vi "user initialization.vi"(8 "error in":errorcluster, 10 "configuration in":refnum<class "control module configuration.lvclass">, 11 "fixed channel runtime in":refnum<class "AppStateMachine runtime.lvclass">) -> (0 "error out":errorcluster, 3 "fixed channel runtime out":refnum<class "AppStateMachine runtime.lvclass">)   [LabVIEW 2017, in "AppStateMachine runtime.lvclass"]
uses:
  AppStateMachine runtime.lvclass
  <vilib>/NI/DCAF/Tag Editor Core/control module/configuration/control module configuration.lvclass
  <vilib>/NI/DCAF/addons/InstructionFrameworkSupport/FPGA_FGV_action.ctl
  <vilib>/userdefined/High Color/nirio_resource_hc.ctl
  StateId.ctl
  State.ctl
  LED_Color.ctl
  AppStateMachine runtime.lvclass/AppStateMachine runtime.ctl
  <vilib>/NI/DCAF/Tag Editor Core/control module/runtime/control module runtime.lvclass
  <vilib>/NI/NI JSONRPC Server Framework/Classes/Server/JSONRPC Server.lvclass
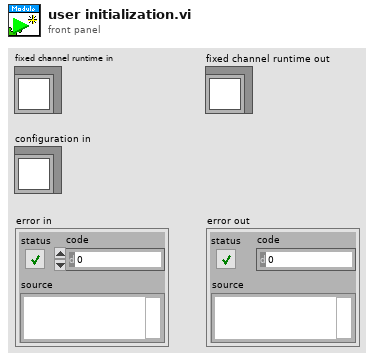
[diagram p1: front panel]
types:
  T1 = typedef "AppStateMachine runtime.lvclass/State.ctl" = cluster{"StateId":T2, "LED_Enable":bool, "LED_BlinksPerCycle":i32, "LED_Color":T3}
  T2 = typedef "AppStateMachine runtime.lvclass/StateId.ctl" = enum16{"Initialize", "Idle", "SafeState", "UnrecoverableSafeState"}
  T3 = typedef "AppStateMachine runtime.lvclass/LED_Color.ctl" = enum16{"Green", "Yellow"}
  T4 = typedef "nirio_resource_hc.ctl" = tag
  T5 = typedef "FPGA_FGV_action.ctl" = enum16{"get FPGA", "set FPGA", "Close"}
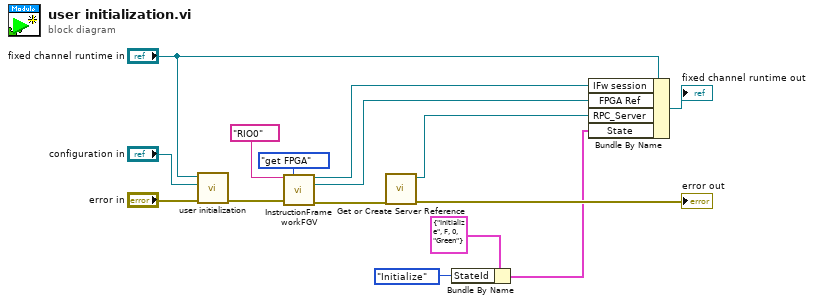
[diagram p0: block diagram]
diagram:
  n1 = call-parent "user initialization.vi"("error in"="error in", "configuration in"="configuration in", "fixed channel runtime in"="fixed channel runtime in") -> ("error out"=w13:errorcluster)  [unwired: 7 in, 1 out]
  n2 = call <vilib>:"InstructionFrameworkFGV.vi"("RIO resource"=T4 "RIO0", "Action"=FPGA_FGV_action."get FPGA", "error in"=w13) -> ("session out"=w10:refnum<class "niInstr FIFO Register Bus v1 Host.lvclass">, "bitfile"=w9:refnum<k20>, "error out"=w6:errorcluster)  [unwired: 10 in]
  n3 = call <vilib>:"Get or Create Server Reference.vi"("error in (no error)"=w6) -> ("error out"=→"error out":errorcluster, "Server Out"=w4:refnum<class "JSONRPC Server.lvclass">)  [unwired: 9 in]
  n4 = Bundle By Name(cluster=T1 {"StateId"=enum."Initialize", "LED_Enable"=FALSE, "LED_BlinksPerCycle"=0, "LED_Color"=enum."Green"} ("State"), "StateId"=StateId."Initialize" ("State")) -> (w1:T1)
  n5 = Bundle By Name(cluster="fixed channel runtime in", "IFw session"=w10, "FPGA Ref"=w9, "RPC_Server"=w4, "State"=w1) -> (→"fixed channel runtime out":refnum<class "AppStateMachine runtime.lvclass">)
